vi "delet.vi"() -> ()   [LabVIEW 2017]
uses:
  <vilib>/addons/database/Connection.llb/DB Tools Open Connec (Path).vi
  <vilib>/addons/database/NI_Database_API.lvlib
panel:
  in  "Station Wise":u16(ring) items=["LH PRE-CONTINUTY ", "RH PRE-CONTINUTY", "LIGHT TEST MACHINE"]
  in  "EXIT":bool
  in  "DELET":bool
  out "barcode":string
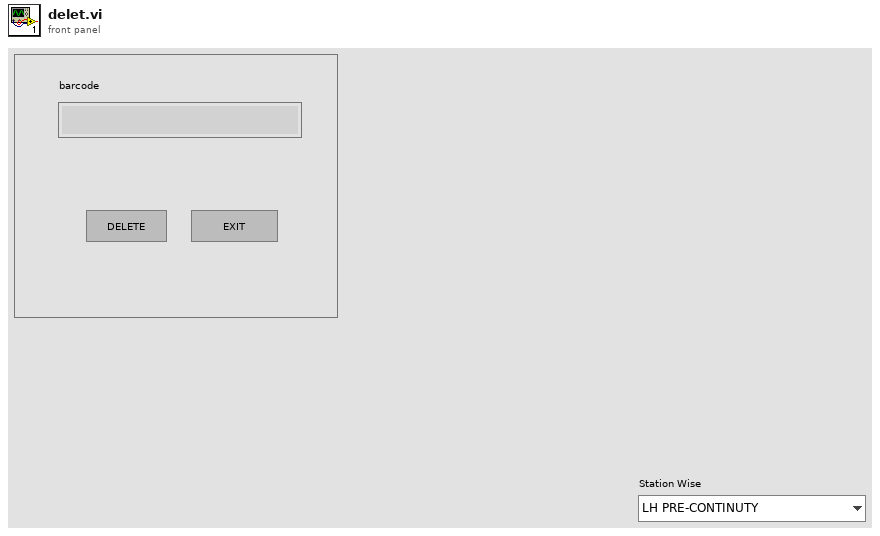
[diagram p1: front panel]
types:
  T1 = typedef "NI_Database_API.lvlib/Conn ObjectReference.ctl" = refnum<k1>
  T2 = enum32{"invalid app kind", "Development System", "Run Time System", "Student Edition", "Embedded LabVIEW", "Evaluation", "Custom"}
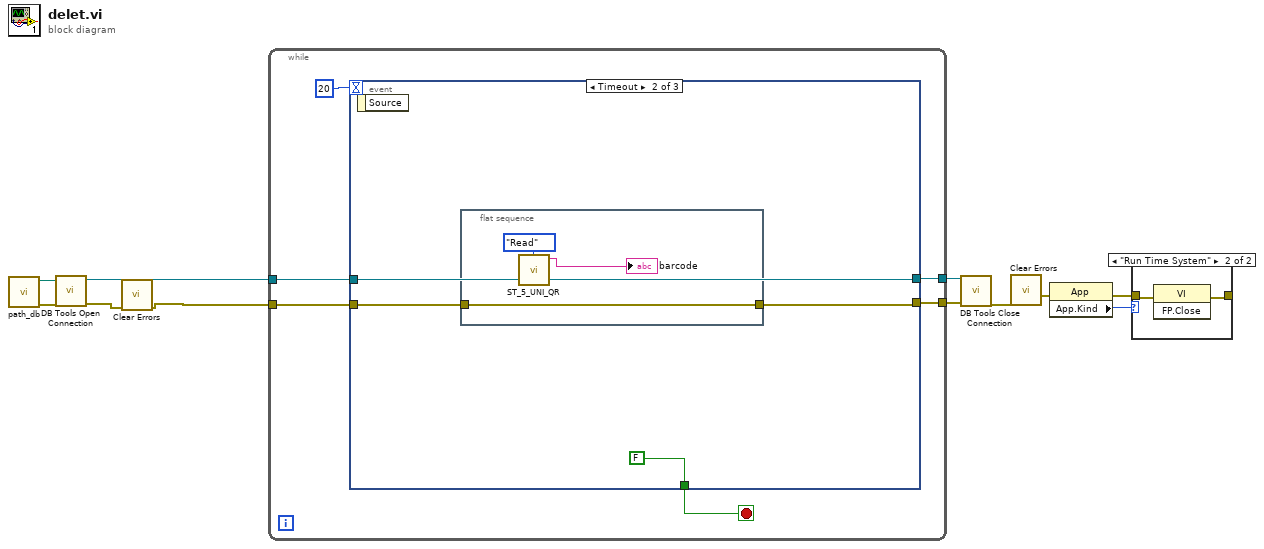
[diagram p0: block diagram]
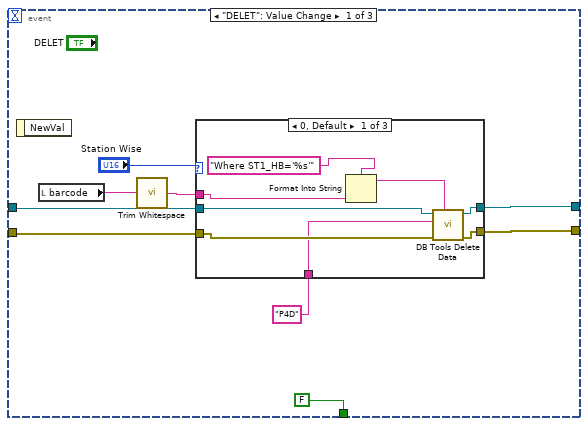
[diagram p3: hidden frame]
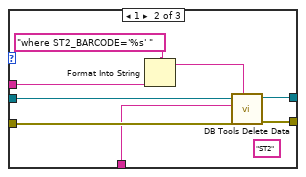
[diagram p4: hidden frame]
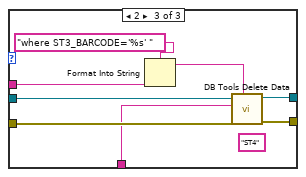
[diagram p5: hidden frame]
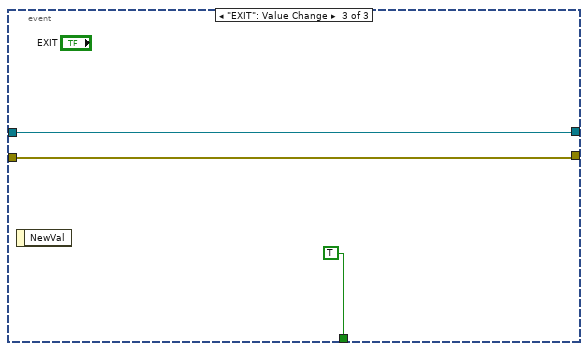
[diagram p6: hidden frame]
diagram:
  n1 = call "path_db.vi"() -> ("error out"=w2:errorcluster, "resulting string"=w1:path)  [unwired: 10 in]
  n2 = call-poly <vilib>:"DB Tools Open Connection.vi"("error in (no error)"=w2, "connection information"=w1) -> ("error out"=w8:errorcluster, "connection reference"=w11:T1)  [unwired: 6 in]
  n3 = call <vilib>:"Clear Errors.vi"("error in (no error)"=w8) -> ("error out"=w7:errorcluster)  [unwired: 5 in, 1 out]
  n4 = while {
    tunnel: w7 -> [w16]
    tunnel: w11 -> [w15]
    tunnel: [w14] -> w10
    tunnel: [w13] -> w9
    stop <- w17 stop-if-true
    n5 = event shown="[1] Timeout" {
      selector: _ -> [_ _ _]
      dyn-events: _ -> [_ _ _]
      timeout: 20 -> [_ _ _]
      tunnel: [FALSE FALSE TRUE] -> w17
      tunnel: w16 -> [w25 w52 w58]
      tunnel: w15 -> [w24 w54 w59]
      tunnel: [w23 w54 w59] -> w14
      tunnel: [w22 w51 w58] -> w13
      event "DELET": Value Change {
        n6 = event-data() -> ()  [unwired: 1 in, 1 out]
        n7 = local read "barcode"() -> (w20:string)
        n8 = call <vilib>:"Trim Whitespace.vi"("string"=w20) -> ("trimmed string"=w19:string)  [unwired: 1 in]
        n9 = case shown="0, Default" "Station Wise" {
          tunnel: w19 -> [w29 w41 w49]
          tunnel: w25 -> [w33 w39 w47]
          tunnel: w24 -> [w32 w38 w46]
          tunnel: [w31 w37 w45] -> w23
          tunnel: [w30 w36 w44] -> w22
          tunnel: "P4D" ("table") -> [w27 w35 w43]
          frame 0, Default {
            n10 = Format Into String(format string="Where ST1_HB='%s'", w29) -> (resulting string=w34:string)  [unwired: 2 in, 1 out]
            n11 = call <vilib>:"DB Tools Delete Data.vi"("condition"=w34, "error in (no error)"=w33, "table"=w27, "connection reference"=w32) -> ("error out"=w30:errorcluster, "connection reference out"=w31:T1)  [unwired: 6 in]
          }
          frame 1 {
            (unwired) "ST2" ("table")
            n12 = Format Into String(format string="where ST2_BARCODE='%s' ", w41) -> (resulting string=w42:string)  [unwired: 2 in, 1 out]
            n13 = call <vilib>:"DB Tools Delete Data.vi"("condition"=w42, "error in (no error)"=w39, "table"=w35, "connection reference"=w38) -> ("error out"=w36:errorcluster, "connection reference out"=w37:T1)  [unwired: 6 in]
          }
          frame 2 {
            (unwired) "ST4" ("table")
            n14 = Format Into String(format string="where ST3_BARCODE='%s' ", w49) -> (resulting string=w50:string)  [unwired: 2 in, 1 out]
            n15 = call <vilib>:"DB Tools Delete Data.vi"("condition"=w50, "error in (no error)"=w47, "table"=w43, "connection reference"=w46) -> ("error out"=w44:errorcluster, "connection reference out"=w45:T1)  [unwired: 6 in]
          }
        }
      }
      event Timeout {
        n16 = event-data() -> ()  [unwired: 1 in, 1 out]
        n17 = flat-sequence {
          tunnel: w52 -> [w57]
          tunnel: [w57] -> w51
          frame #0 {
            n18 = call "ST_5_UNI_QR.vi"("Enum"=enum16{"Read", "Write"}."Read") -> ("LB QR ST 5"=→"barcode":string)  [unwired: 9 in, 1 out]
          }
        }
      }
      event "EXIT": Value Change {
        n19 = event-data() -> ()  [unwired: 1 in, 1 out]
      }
    }
  }
  n20 = call <vilib>:"DB Tools Close Connection.vi"("error in (no error)"=w9, "connection reference"=w10) -> ("error out"=w6:errorcluster)  [unwired: 5 in]
  n21 = call <vilib>:"Clear Errors.vi"("error in (no error)"=w6) -> ("error out"=w4:errorcluster)  [unwired: 5 in, 1 out]
  n22 = property class="App"(error in=w4) -> (error out=w3:errorcluster, "App.Kind"=w5:T2)  [unwired: 1 in, 1 out]
  n23 = case shown="\"Run Time System\"" w5 {
    tunnel: w3 -> [w61 w63]
    tunnel: [w61 w62] -> _
    frame Default {
    }
    frame "Run Time System" {
      n24 = invoke class="VI" method="FP.Close"(error in=w63) -> (error out=w62:errorcluster)  [unwired: 2 in, 2 out]
    }
  }
